vi "Set Or get ActiveCell Bk Color.vi"(8 "error in (no error)":errorcluster caption="错误输入（无错误）", 9 "Mode":T1, 10 "BK Color In":u32(colorbox), 11 "Table Ref In":refnum<vi>) -> (0 "error out":errorcluster caption="错误输出", 2 "BK Color Out":u32(colorbox), 3 "Table Ref Out":refnum<vi>)   [LabVIEW 2012, in "Table Tool.lvlib"]
uses:
  Table Tool.lvlib
  GetOrSet.ctl
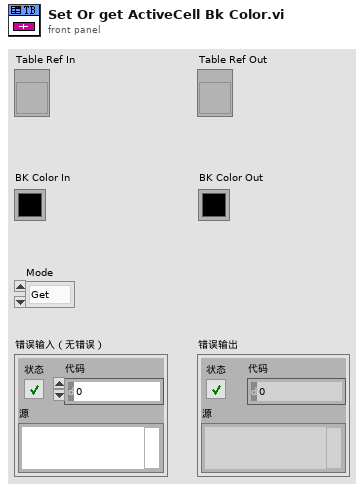
[diagram p1: front panel]
types:
  T1 = typedef "Table Tool.lvlib/GetOrSet.ctl" = enum16{"Get", "Set"}
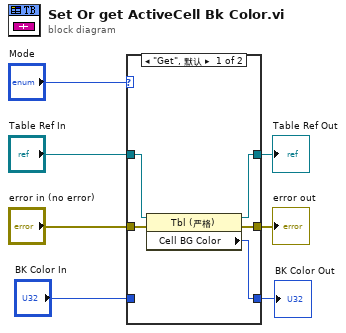
[diagram p0: block diagram]
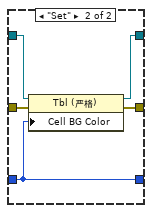
[diagram p2: hidden frame]
diagram:
  n1 = case shown="\"Get\", 默认" "Mode" {
    tunnel: "Table Ref In" -> [w12 w16]
    tunnel: "error in (no error)" -> [w11 w17]
    tunnel: [w10 w14] -> w4
    tunnel: [w9 w15] -> w3
    tunnel: [w8 w13] -> w1
    tunnel: "BK Color In" -> [_ w13]
    frame "Get", Default {
      n2 = property class="Tbl (严格)"(reference=w12, error in=w11) -> (reference out=w9:refnum<vi>, error out=w10:errorcluster, "Cell BG Color"=w8:u32)
    }
    frame "Set" {
      n3 = property class="Tbl (严格)"(reference=w16, error in=w17, "Cell BG Color"=w13) -> (reference out=w15:refnum<vi>, error out=w14:errorcluster)
    }
  }
  "Table Ref Out" <- w3
  "error out" <- w4
  "BK Color Out" <- w1
